vi "dIMU_Gyro_Poly.vi"   [LabVIEW 2010]
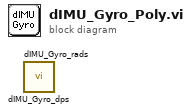
[diagram p0: block diagram]
diagram:
  n1 = call "dIMU_Gyro_rads.vi"() -> ()  [unwired: 8 in, 4 out]
  n2 = call "dIMU_Gyro_dps.vi"() -> ()  [unwired: 8 in, 4 out]
